vi "Constants.vi"() -> (1 "PPL Name":string="main.vi", 3 "HelperMain Name":string="main.vi", 4 "Root Path":path, 6 "HelperMain path":path, 8 "HelperExecutable path":path, 10 "HelperProject path":path, 15 "TestPPL Path":path)   [LabVIEW 2016, in "DronaTest.lvlib"]
uses:
  DronaTest.lvlib
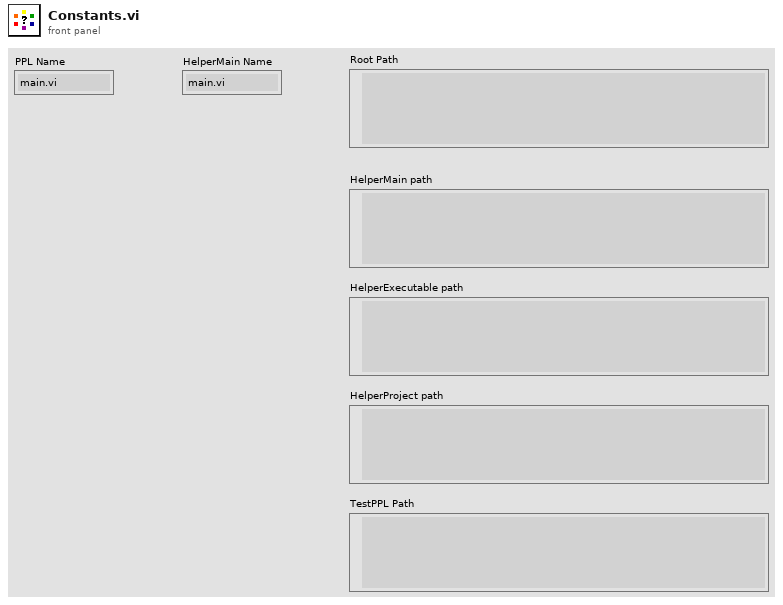
[diagram p1: front panel]
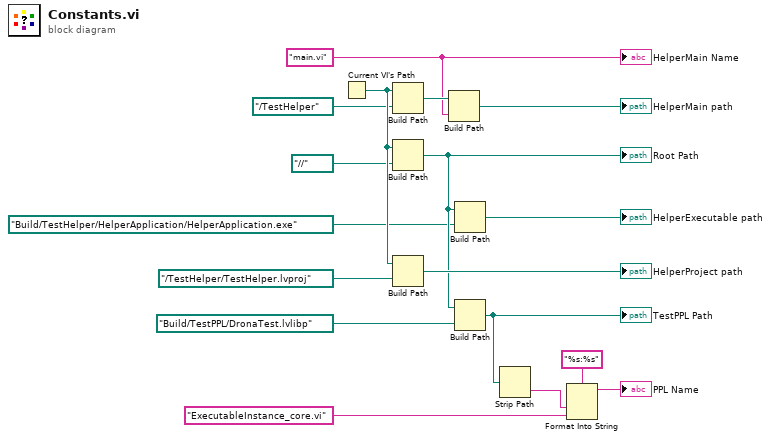
[diagram p0: block diagram]
diagram:
  w14 = "main.vi" ("name or relative path")
  n1 = Current VI's Path() -> (path=w12:path)
  n2 = Build Path(base path=w12, name or relative path=path "../TestHelper" ("appended path")) -> (appended path=w15:path)
  n3 = Build Path(base path=w12, name or relative path=path "../../.." ("appended path")) -> (appended path=w11:path)
  "Root Path" <- w11
  n4 = Build Path(base path=w12, name or relative path=path "../TestHelper/TestHelper.lvproj" ("appended path")) -> (appended path=→"HelperProject path":path)
  n5 = Build Path(base path=w15, name or relative path=w14) -> (appended path=→"HelperMain path":path)
  n6 = Build Path(base path=w11, name or relative path=path "Build/TestHelper/HelperApplication/HelperApplication.exe" ("appended path")) -> (appended path=→"HelperExecutable path":path)
  n7 = Build Path(base path=w11, name or relative path=path "Build/TestPPL/DronaTest.lvlibp" ("appended path")) -> (appended path=w10:path)
  "TestPPL Path" <- w10
  n8 = Strip Path(path=w10) -> (name=w9:string)  [unwired: 1 out]
  n9 = Format Into String(format string="%s:%s", w9, "ExecutableInstance_core.vi" ("PPL Name")) -> (resulting string=→"PPL Name":string)  [unwired: 2 in, 1 out]
  "HelperMain Name" <- w14
